vi "Add NI-XNET CAN Hardware_Add CAN.vi"(7 "SysDef Ref":T7, 8 "error in (no error)":errorcluster, 9 "CAN Settings":T1={"Name"="", "Database Name"="", "PortNumber"=0, "ClusterName"="", "BaudRate"=500000, "InlineIncoming"=FALSE, "IncomingRate"=100, "InlineOutgoing"=FALSE, "OutgoingRate"=100, "Termination"=0, "Echo"=FALSE, "InputStreamQueueSize"=120000, "CANBusOff"=FALSE, "CANBusOffRate"=1, "TransceiverType"=0, "TransmitOrderType"=0, "Cyclic Frames"=[], "Outgoing Frames"=[], "Incoming Frames"=[], "Log Files"=[]} {"Log Files"."Operation" items=["ContinueLoggingInNewFile", "StopLogging"]; "Log Files"."LimitType" items=["Footprint", "Time"]; "Log Files"."TriggerType" items=["StartLoggingOnNonZero", "StartLoggingOnZero", "EnableLoggingWhenTriggerIsZero", "EnableLoggingWhenTriggerIsNonZero"]; "Log Files"."Filter" items=["LogEntireBusTraffic", "ExcludeFrameIDs", "IncludeFrameIDs"]; "Log Files"."DataLoggingFileType" items=["TDMS", "NCL"]; "TransmitOrderType" items=["AsSubmitted", "ByIdentifier"]; "TransceiverType" items=["HS", "LS", "SW"]; "Termination" items=["Off", "On"]; "Outgoing Frames"."Phase" items=["Unchanged", "Reset"]; "Outgoing Frames"."TriggerType" items=["ChannelValueChange", "TriggerChannelNotZero", "ChannelValueChangeOrTriggerChannelNotZero"]}, 11 "CAN Ref":refnum<k24>) -> (0 "error out":errorcluster, 3 "CAN Ref Out":refnum<k24>)   [LabVIEW 2019, in "Simple SysDef API.lvlib"]
uses:
  <userlib>/SimpleSysDef/Simple SysDef API.lvlib
  NationalInstruments.VeriStand.SystemDefinitionAPI
  <userlib>/SimpleSysDef/_SubVIs/System Definition Reference.ctl
  <userlib>/SimpleSysDef/_SubVIs/Add NI-XNET CAN Hardware_Port Settings.ctl
  <userlib>/SimpleSysDef/_SubVIs/Add NI-XNET CAN Hardware_Periodic Frame Settings.ctl
  <userlib>/SimpleSysDef/_SubVIs/Add NI-XNET CAN Hardware_Frame Settings.ctl
  <userlib>/SimpleSysDef/_SubVIs/Add NI-XNET CAN Hardware_Signal Settings.ctl
  <userlib>/SimpleSysDef/_SubVIs/Add NI-XNET CAN Hardware_Sporadic Frame Settings.ctl
  <userlib>/SimpleSysDef/_SubVIs/Add NI-XNET CAN Hardware_Add Log File_Settings.ctl
  NationalInstruments.VeriStand
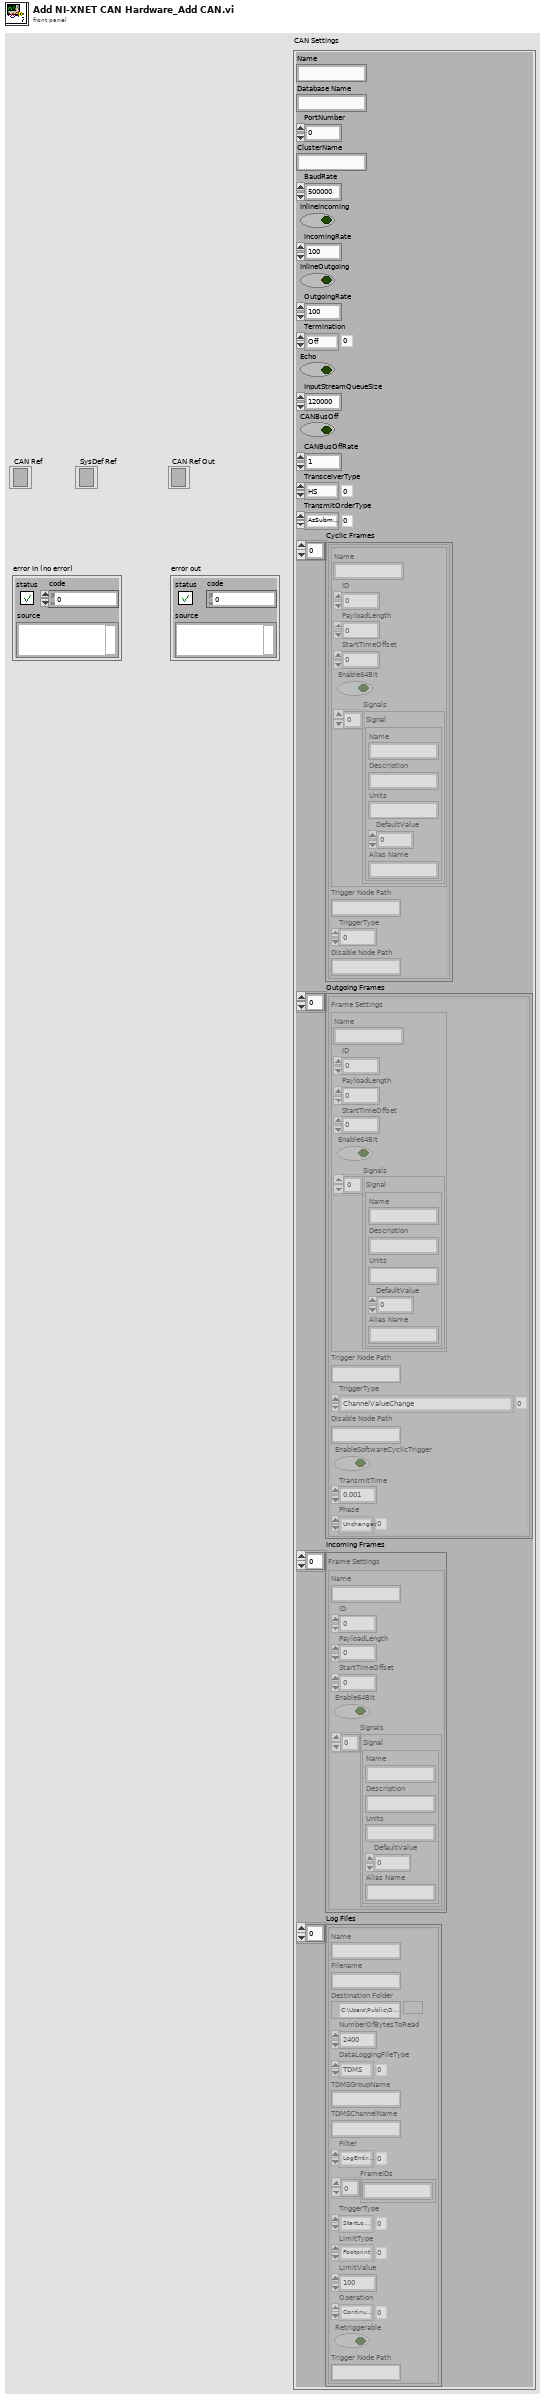
[diagram p1: front panel]
types:
  T1 = typedef "Simple SysDef API.lvlib/Add NI-XNET CAN Hardware_Port Settings.ctl" = cluster{"Name":string, "Database Name":string, "PortNumber":u16, "ClusterName":string, "BaudRate":u32, "InlineIncoming":bool, "IncomingRate":u32, "InlineOutgoing":bool, "OutgoingRate":u32, "Termination":i32, "Echo":bool, "InputStreamQueueSize":u32, "CANBusOff":bool, "CANBusOffRate":u32, "TransceiverType":i32, "TransmitOrderType":i32, "Cyclic Frames":T2[], "Outgoing Frames":T5[], "Incoming Frames":T3[], "Log Files":T6[]}
  T2 = typedef "Simple SysDef API.lvlib/Add NI-XNET CAN Hardware_Periodic Frame Settings.ctl" = cluster{"Frame Settings":T3, "Trigger Node Path":string, "TriggerType":i32, "Disable Node Path":string}
  T3 = typedef "Simple SysDef API.lvlib/Add NI-XNET CAN Hardware_Frame Settings.ctl" = cluster{"Name":string, "ID":u32, "PayloadLength":u32, "StartTimeOffset":dbl, "Enable64Bit":bool, "Signals":T4[]}
  T4 = typedef "Simple SysDef API.lvlib/Add NI-XNET CAN Hardware_Signal Settings.ctl" = cluster{"Name":string, "Description":string, "Units":string, "DefaultValue":dbl, "Alias Name":string}
  T5 = typedef "Simple SysDef API.lvlib/Add NI-XNET CAN Hardware_Sporadic Frame Settings.ctl" = cluster{"Frame Settings":T3, "Trigger Node Path":string, "TriggerType":i32, "Disable Node Path":string, "EnableSoftwareCyclicTrigger":bool, "TransmitTime":dbl, "Phase":i32}
  T6 = typedef "Simple SysDef API.lvlib/Add NI-XNET CAN Hardware_Add Log File_Settings.ctl" = cluster{"Name":string, "Filename":string, "Destination Folder":path, "NumberOfBytesToRead":u32, "DataLoggingFileType":i32, "TDMSGroupName":string, "TDMSChannelName":string, "Filter":i32, "FrameIDs":string[], "TriggerType":i32, "LimitType":i32, "LimitValue":u32, "Operation":i32, "Retriggerable":bool, "Trigger Node Path":string}
  T7 = typedef "Simple SysDef API.lvlib/System Definition Reference.ctl" = refnum<k24>
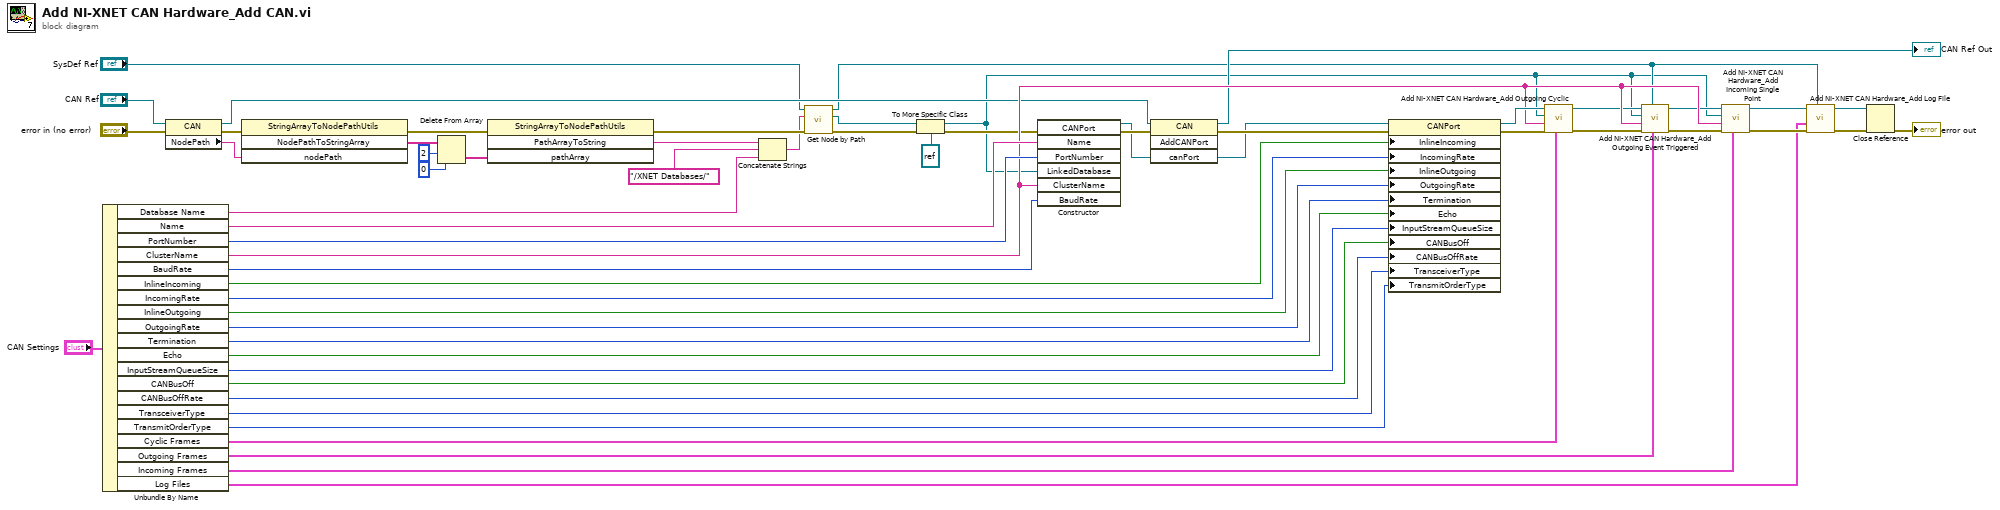
[diagram p0: block diagram]
diagram:
  n1 = Unbundle By Name("CAN Settings") -> ("Database Name"=w7:string, "Name"=w52:string, "PortNumber"=w51:u16, "ClusterName"=w36:string, "BaudRate"=w50:u32, "InlineIncoming"=w49:bool, "IncomingRate"=w48:u32, "InlineOutgoing"=w47:bool, "OutgoingRate"=w46:u32, "Termination"=w45:i32, "Echo"=w44:bool, "InputStreamQueueSize"=w43:u32, "CANBusOff"=w42:bool, "CANBusOffRate"=w41:u32, "TransceiverType"=w40:i32, "TransmitOrderType"=w39:i32, "Cyclic Frames"=w30:T2[], "Outgoing Frames"=w29:T5[], "Incoming Frames"=w28:T3[], "Log Files"=w27:T6[])
  n2 = property class="CAN"(reference="CAN Ref", error in="error in (no error)") -> (reference out=w20:refnum<k24>, error out=w18:errorcluster, "NodePath"=w19:string)
  n3 = invoke class="StringArrayToNodePathUtils" method="NodePathToStringArray"(error in=w18, "nodePath"=w19) -> (error out=w14:errorcluster, "NodePathToStringArray"=w17:string[])  [unwired: 2 in, 2 out]
  n4 = Delete From Array(array=w17, length=2, index=0) -> (deleted portion=w1:string[])  [unwired: 1 out]
  n5 = invoke class="StringArrayToNodePathUtils" method="PathArrayToString"(error in=w14, "pathArray"=w1) -> (error out=w13:errorcluster, "PathArrayToString"=w12:string)  [unwired: 2 in, 2 out]
  n6 = Concatenate Strings(w12, "/XNET Databases/" ("string"), w7) -> (w10:string)
  n7 = call <userlib>:"Get Node by Path.vi"("error in (no error)"=w13, "System Definition Node Path"=w10, "SysDef Ref"="SysDef Ref") -> ("error out"=w5:errorcluster, "Node Ref"=w3:refnum<k24>, "SysDef Ref Out"=w8:T7)  [unwired: 6 in]
  n8 = To More Specific Class(target class=refnum<k24> refnum ("Node Ref"), reference=w3, error in=w5) -> (specific class reference=w2:refnum<k24>, error out=w4:errorcluster)
  n9 = constructor class="CANPort"(error in=w4, "Name"=w52, "PortNumber"=w51, "LinkedDatabase"=w2, "ClusterName"=w36, "BaudRate"=w50) -> (reference out=w55:refnum<k24>, error out=w57:errorcluster)  [unwired: 2 in, 6 out]
  n10 = invoke class="CAN" method="AddCANPort"(reference=w20, error in=w57, "canPort"=w55) -> (reference out=→"CAN Ref Out":refnum<k24>, error out=w56:errorcluster)  [unwired: 1 in, 2 out]
  n11 = property class="CANPort"(reference=w55, error in=w56, "InlineIncoming"=w49, "IncomingRate"=w48, "InlineOutgoing"=w47, "OutgoingRate"=w46, "Termination"=w45, "Echo"=w44, "InputStreamQueueSize"=w43, "CANBusOff"=w42, "CANBusOffRate"=w41, "TransceiverType"=w40, "TransmitOrderType"=w39) -> (reference out=w38:refnum<k24>, error out=w37:errorcluster)
  n12 = call <userlib>:"Add NI-XNET CAN Hardware_Add Outgoing Cyclic.vi"("Cyclic Frames"=w30, "error in (no error)"=w37, "ClusterName"=w36, "Owning Database"=w2, "CAN Port"=w38) -> ("error out"=w35:errorcluster, "CAN Port out"=w34:refnum<k24>)  [unwired: 5 in]
  n13 = call <userlib>:"Add NI-XNET CAN Hardware_Add Outgoing Event Triggered.vi"("Sporadic Frames"=w29, "SysDef Ref"=w8, "error in (no error)"=w35, "ClusterName"=w36, "Owning Database"=w2, "CAN Port"=w34) -> ("error out"=w33:errorcluster, "CAN Port out"=w32:refnum<k24>)  [unwired: 4 in]
  n14 = call <userlib>:"Add NI-XNET CAN Hardware_Add Incoming Single Point.vi"("Single Point Frames"=w28, "error in (no error)"=w33, "ClusterName"=w36, "Owning Database"=w2, "CAN Port"=w32) -> ("error out"=w54:errorcluster, "CAN Port out"=w53:refnum<k24>)  [unwired: 5 in]
  n15 = call <userlib>:"Add NI-XNET CAN Hardware_Add Log File.vi"("SysDef Ref"=w8, "error in (no error)"=w54, "Log Files"=w27, "CAN Port Ref"=w53) -> ("error out"=w25:errorcluster, "CAN Port Ref out"=w26:refnum<k24>)  [unwired: 6 in]
  n16 = Close Reference(reference=w26, error in (no error)=w25) -> (error out=→"error out":errorcluster)
